vi "lock-in_send_analysis.vi"(7 "order":T2(ring)=enum."Data sent to host", 8 "data sent back":u8(ring) items=["LI", "average"], 9 "dt/tau":fxp<+,32,0>, 10 "Voltage range":u16(ring) items=["10V", "5V", "1V"], 11 "FPGA VI Reference In":T1) -> (3 "FPGA VI Reference Out":T1)   [LabVIEW 2013]
uses:
  fpga-bitfile-ref.ctl
  <vilib>/Utility/error.llb/Error Cluster From Error Code.vi
  <vilib>/rvi/errors/niLvFpgaAdjustHostInterfaceError.vi
  <vilib>/rvi/interface/nirviReadWriteControl/nirviReadWriteControl.xnode
  FPGA Bitfiles/fpga-clean1_FPGATarget_FPGAMAINlock-in_FC21E42C.lvbitx
  NiFpgaLv.dll
panel:
  out "error out":errorcluster
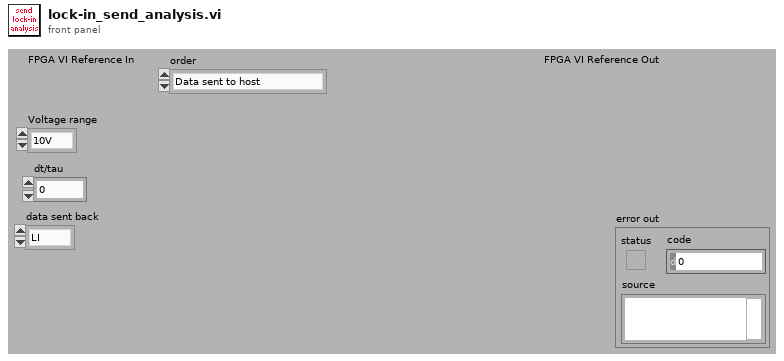
[diagram p1: front panel]
types:
  T1 = typedef "fpga-bitfile-ref.ctl" = refnum<k20>
  T2 = enum8{"NULL", "Data sent to host", "dt/tau", "Voltage range"}
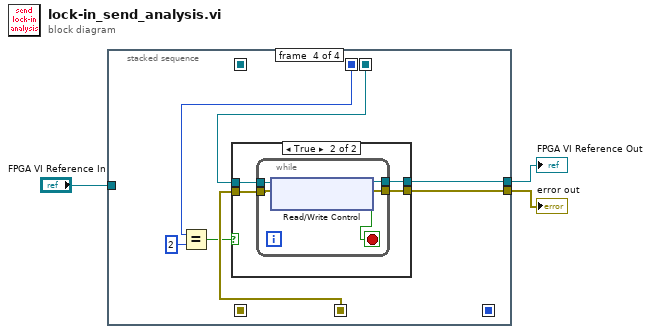
[diagram p0: block diagram]
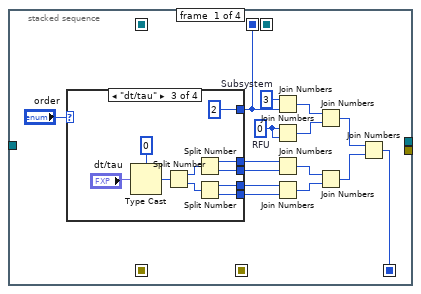
[diagram p2: hidden frame]
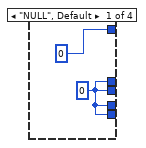
[diagram p3: hidden frame]
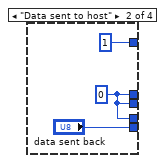
[diagram p4: hidden frame]
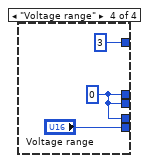
[diagram p5: hidden frame]
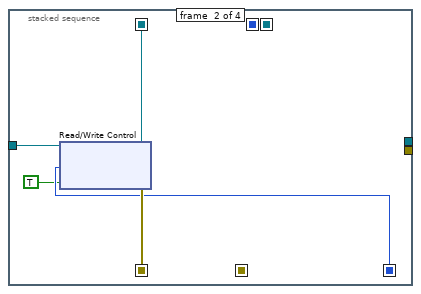
[diagram p6: hidden frame]
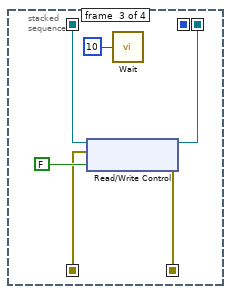
[diagram p7: hidden frame]
diagram:
  n1 = stacked-sequence {
    seq-local: [w6 _ _ _] -> [_ w39 _ _]
    seq-local: [w4 _ _ _] -> [_ _ _ w48]
    seq-local: [_ w41 _ _] -> [_ _ w46 _]
    seq-local: [_ w40 _ _] -> [_ _ w43 _]
    seq-local: [_ _ w45 _] -> [_ _ _ w54]
    seq-local: [_ _ w44 _] -> [_ _ _ w53]
    tunnel: "FPGA VI Reference In" -> [_ w37 _ _]
    tunnel: [_ _ _ w52] -> w1
    tunnel: [_ _ _ w51] -> w2
    frame #0 {
      w9 = u8 3  # Subsystem
      w18 = u8 0  # RFU
      n2 = case shown="\"dt/tau\"" "order" {
        tunnel: [w20 w23 w28 w35] -> w14
        tunnel: [w20 w23 w29 w35] -> w16
        tunnel: [w20 w23 w30 w35] -> w17
        tunnel: [w20 "data sent back" w27 "Voltage range"] -> w15
        tunnel: [u8 0 ("order") u8 1 ("order") u8 2 ("order") u8 3 ("order")] -> w4
        frame "NULL", Default {
          w20 = u8 0
        }
        frame "Data sent to host" {
          w23 = u8 0
        }
        frame "dt/tau" {
          n3 = Type Cast(type=u32 0 ("order"), x="dt/tau") -> (*(type *) &x=w26:u32)
          n4 = Split Number(x=w26) -> (hi(x)=w31:u16, lo(x)=w32:u16)
          n5 = Split Number(x=w31) -> (hi(x)=w30:u8, lo(x)=w29:u8)
          n6 = Split Number(x=w32) -> (hi(x)=w28:u8, lo(x)=w27:u8)
        }
        frame "Voltage range" {
          w35 = u8 0 ("order")
        }
      }
      n7 = Join Numbers(hi=w9, lo=w4) -> ((hi.lo)=w10:u16)
      n8 = Join Numbers(hi=w18, lo=w18) -> ((hi.lo)=w11:u16)
      n9 = Join Numbers(hi=w17, lo=w16) -> ((hi.lo)=w12:u16)
      n10 = Join Numbers(hi=w14, lo=w15) -> ((hi.lo)=w13:u32)
      n11 = Join Numbers(hi=w10, lo=w11) -> ((hi.lo)=w7:u32)
      n12 = Join Numbers(hi=w12, lo=w13) -> ((hi.lo)=w8:u64)
      n13 = Join Numbers(hi=w7, lo=w8) -> ((hi.lo)=w6:u64)
    }
    frame #1 {
      n14 = xnode "Read/Write Control"("FPGA VI Reference In"=w37, "order in"=w39, "order Xmitted"=TRUE) -> ("FPGA VI Reference Out"=w41:T1, "error out"=w40:errorcluster)  [unwired: 1 in]
    }
    frame #2 {
      n15 = xnode "Read/Write Control"("FPGA VI Reference In"=w46, "error in"=w43, "order Xmitted"=FALSE) -> ("FPGA VI Reference Out"=w45:T1, "error out"=w44:errorcluster)
      n16 = call "Wait"("Count(mSec)"=u32 10) -> ()  [unwired: 1 out]
    }
    frame #3 {
      n17 = Equal?(x=w48, y=u8 2) -> (x = y?=w50:bool)
      n18 = case shown="True" w50 {
        tunnel: w54 -> [w56 w60]
        tunnel: w53 -> [w55 w59]
        tunnel: [w56 w58] -> w52
        tunnel: [w55 w57] -> w51
        frame False {
        }
        frame True {
          n19 = while {
            tunnel: w60 -> [w65]
            tunnel: w59 -> [w64]
            tunnel: [w63] -> w58
            tunnel: [w62] -> w57
            stop <- w61 stop-if-true
            n20 = xnode "Read/Write Control"("FPGA VI Reference In"=w65, "error in"=w64) -> ("FPGA VI Reference Out"=w63:T1, "error out"=w62:errorcluster, "move bus ready"=w61:bool)
          }
        }
      }
    }
  }
  "error out" <- w2
  "FPGA VI Reference Out" <- w1
